vi "Write Size of experimeents.vi"(8 "error in (no error)":errorcluster, 9 "Temp":bool, 10 "Size of experimeents":cluster{"X pixels":i32, "Y pixels":i32}[](array[cluster]), 11 "Experiment_merged in":refnum<class "Experiment_merged.lvclass">) -> (0 "error out":errorcluster, 3 "Experiment_merged out":refnum<class "Experiment_merged.lvclass">)   [LabVIEW 2018, in "Experiment_merged.lvclass"]
uses:
  Experiment_merged.lvclass
  Experiment_merged.lvclass/Experiment_merged.ctl
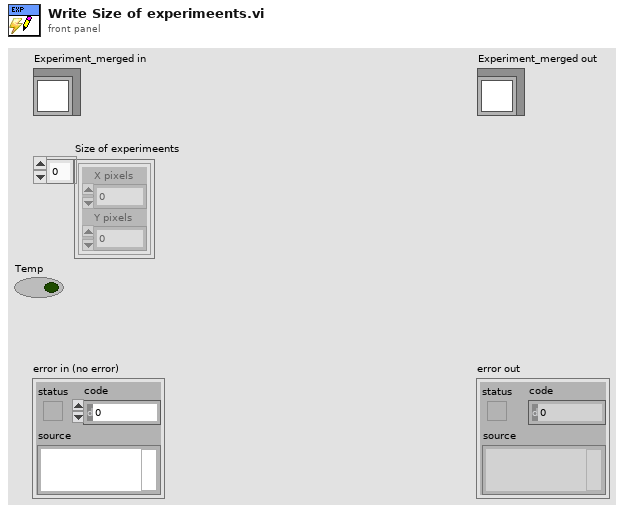
[diagram p1: front panel]
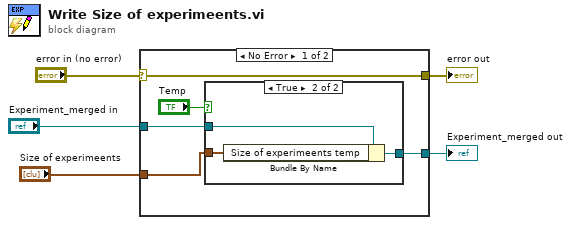
[diagram p0: block diagram]
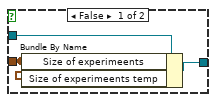
[diagram p2: hidden frame]
diagram:
  n1 = case shown="No Error" "error in (no error)" {
    selector: "error in (no error)" -> [w10 w17]
    tunnel: [w10 w17] -> w4
    tunnel: [w8 w18] -> w2
    tunnel: "Experiment_merged in" -> [w9 w18]
    tunnel: "Size of experimeents" -> [w7 _]
    frame No Error {
      n2 = case shown="True" "Temp" {
        tunnel: w9 -> [w13 w16]
        tunnel: [w12 w15] -> w8
        tunnel: w7 -> [w11 w14]
        frame False {
          n3 = Bundle By Name(cluster=w13, "Size of experimeents"=w11, "Size of experimeents temp"=w11) -> (w12:refnum<class "Experiment_merged.lvclass">)
        }
        frame True {
          n4 = Bundle By Name(cluster=w16, "Size of experimeents temp"=w14) -> (w15:refnum<class "Experiment_merged.lvclass">)
        }
      }
    }
    frame Error {
    }
  }
  "error out" <- w4
  "Experiment_merged out" <- w2
